vi "Signal IO (SubVI)_SIL.vi"(4 "ROV string":string="34.5,,,,$56.3,34.556,,,,$67.9", 5 "NAVI string":string="!init;50;70;0;0;;;;") -> (1 "dvl_m":dbl[](array[numeric]), 10 "ROV OK":string, 12 "Navi OK":string, 13 "Signals out":dbl[](array[numeric]), 15 "port1 a":string, 16 "port 2 a":string)   [LabVIEW 2014]
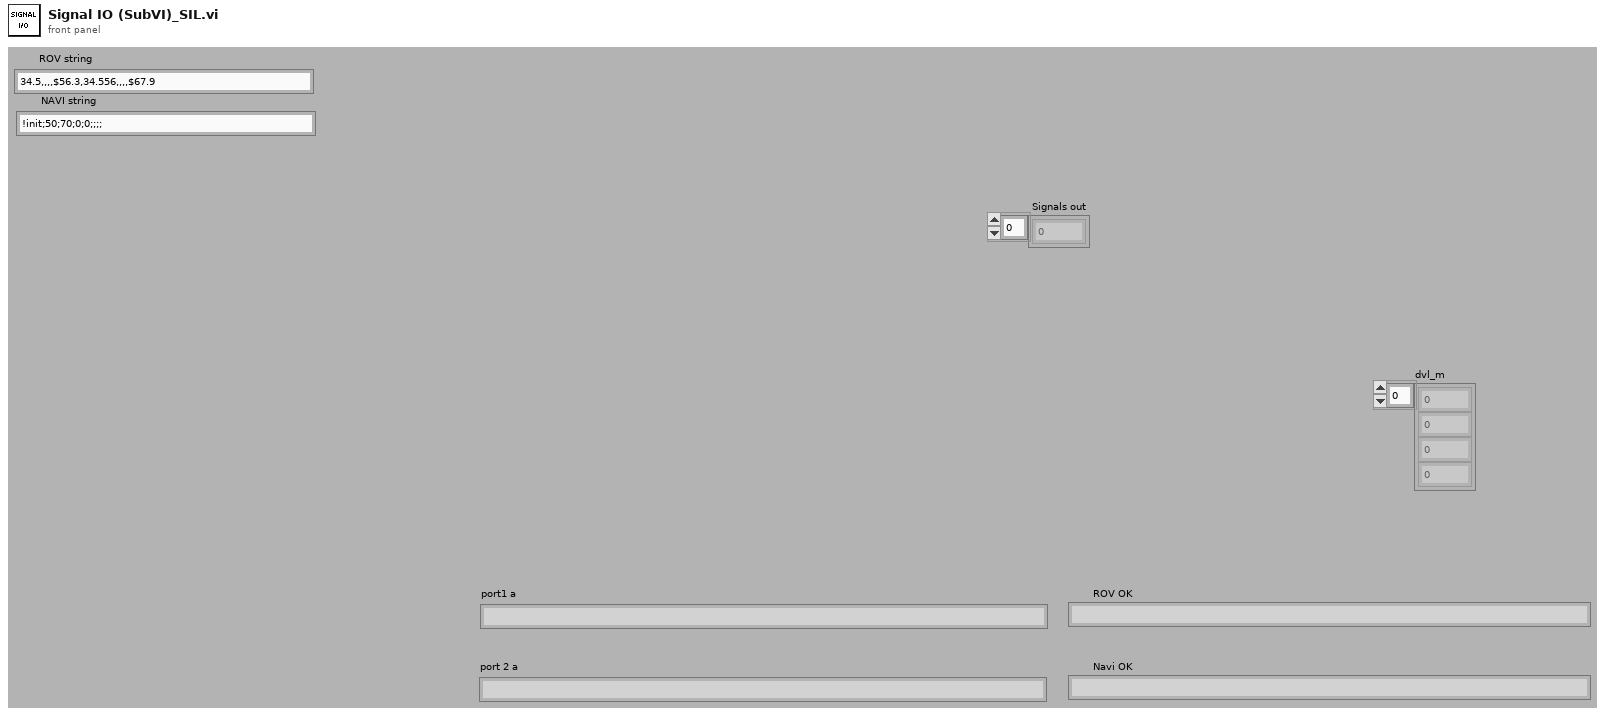
[diagram p1: front panel]
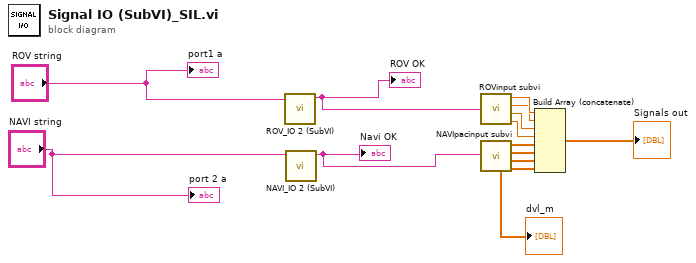
[diagram p0: block diagram]
diagram:
  n1 = call "ROV_IO 2 (SubVI).vi"("ROV string"="ROV string") -> ("ROV OK"=w13:string)  [unwired: 10 in]
  "ROV OK" <- w13
  n2 = call "NAVI_IO 2 (SubVI).vi"("NAVI string"="NAVI string") -> ("NAVI OK"=w14:string)  [unwired: 10 in]
  "Navi OK" <- w14
  n3 = call "ROVinput subvi.vi"("String"=w13) -> ("depth"=w6:dbl, "altitude"=w3:dbl, "heading"=w7:dbl, "yaw rate"=w8:dbl)
  n4 = call "NAVIpacinput subvi.vi"("String"=w14) -> ("Pos_s"=→"dvl_m":dbl[], "a_dvl"=w12:dbl[], "vw_dvl"=w11:dbl[], "vb_dvl"=w10:dbl[], "NED_tp"=w9:dbl[])  [unwired: 1 out]
  n5 = Build Array (concatenate)(w6, w3, w7, w8, w9, w10, w11, w12) -> (→"Signals out":dbl[])
  "port1 a" <- "ROV string"
  "port 2 a" <- "NAVI string"
